vi "DataSockets Open.vi"(8 "error IO":errorcluster, 9 "mode":T1(ring), 10 "Variables":string[](array[string]), 11 "Main Path":string) -> (0 "error out":errorcluster, 3 "Array":refnum<k13>[](array[refnum]))   [LabVIEW 2014]
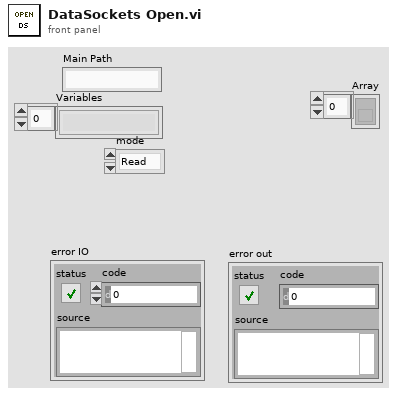
[diagram p1: front panel]
types:
  T1 = enum16{"Read", "Write", "ReadWrite", "BufferedRead", "BufferedReadWrite"}
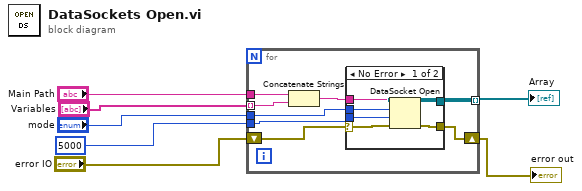
[diagram p0: block diagram]
diagram:
  n1 = for {
    tunnel: "Main Path" -> [w15]
    tunnel: "Variables" -> [w14] mode=indexing
    tunnel: [w12] -> w7 mode=indexing
    shift-right: [w11] -> w4
    shift-left: "error IO" -> [w10]
    tunnel: 5000 ("ms timeout (10000)") -> [w9]
    tunnel: "mode" -> [w8]
    n2 = Concatenate Strings(w15, w14) -> (w13:string)
    n3 = case shown="No Error" w10 {
      selector: w10 -> [w18 w22]
      tunnel: w13 -> [w21 _]
      tunnel: [w20 _] -> w12
      tunnel: [w19 w22] -> w11
      tunnel: w9 -> [w17 _]
      tunnel: w8 -> [w16 _]
      frame No Error {
        n4 = DataSocket Open(8:w18, 9:w17, 10:w16, 11:w21) -> (0:w19:errorcluster, 3:w20:refnum<k13>)
      }
      frame Error {
      }
    }
  }
  "Array" <- w7
  "error out" <- w4
